vi "Referential Leaves to Objects.vi"(11 "Reference Items":T1(array[cluster])) -> (3 "Reference Objects":refnum<class "Referential.lvclass">[](array[class]))   [LabVIEW 2019, in "ParseGDSII.lvclass"]
uses:
  ParseGDSII.lvclass
  Elements/Referential.lvclass
  06f77329-d20e-40e9-99c9-cf91113c5fcf.vi/492f4e88-b7c6-4100-97d4-f1e35eb10a82.vi
  <vilib>/Utility/Debug Log/Display.vi
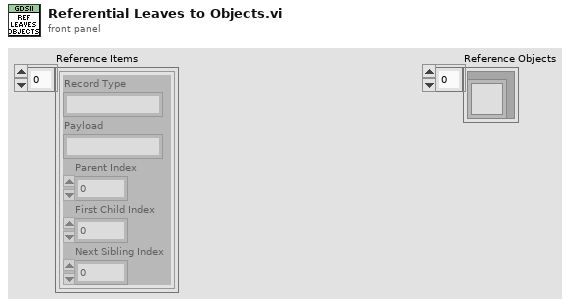
[diagram p1: front panel]
types:
  T1 = cluster{"Record Type":string, "Payload":string, "Parent Index":i32, "First Child Index":i32, "Next Sibling Index":i32}[]
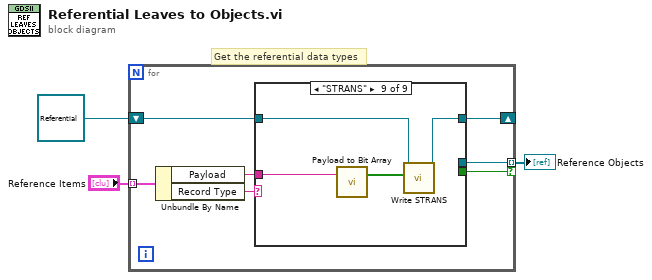
[diagram p0: block diagram]
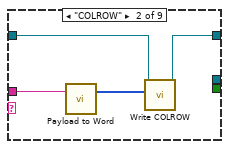
[diagram p3: hidden frame]
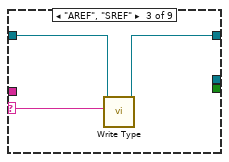
[diagram p4: hidden frame]
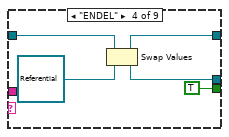
[diagram p5: hidden frame]
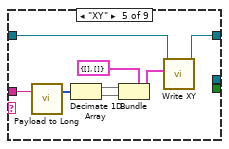
[diagram p6: hidden frame]
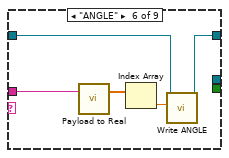
[diagram p7: hidden frame]
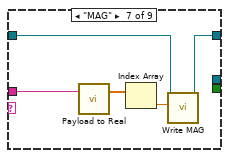
[diagram p8: hidden frame]
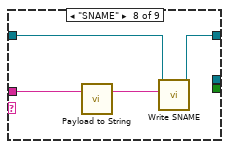
[diagram p9: hidden frame]
diagram:
  # "Get the referential data types"
  n1 = for {
    tunnel: "Reference Items" -> [w10] mode=indexing
    tunnel: [w5] -> w1 mode=indexing if=w4
    shift-right: [w7] -> _
    shift-left: refnum<class "Referential.lvclass"> refnum ("Referential.lvclass") -> [w6]
    n2 = Unbundle By Name(w10) -> ("Payload"=w9:string, "Record Type"=w8:string)
    n3 = case shown="\"STRANS\"" w8 {
      selector: w8 -> [_ _ w16 _ _ _ _ _ _]
      tunnel: w9 -> [_ w15 _ _ w26 w32 w40 w43 w47]
      tunnel: [w11 w12 w18 w20 w25 w35 w38 w45 w48] -> w7
      tunnel: w6 -> [w11 w13 w17 w21 w24 w36 w39 w44 w49]
      tunnel: [_ _ _ w22 _ _ _ _ _] -> w5
      tunnel: [_ _ _ TRUE _ _ _ _ _] -> w4
      frame Default {
      }
      frame "COLROW" {
        n4 = call "Payload to Word.vi"("Payload"=w15) -> ("Word"=w14:i16[])  [unwired: 2 in]
        n5 = call-dynamic "Write COLROW.vi"("COLROW"=w14, "Referential in"=w13) -> ("Referential out"=w12:refnum<class "Referential.lvclass">)  [unwired: 8 in, 1 out]
      }
      frame "AREF", "SREF" {
        n6 = call-dynamic "Write Type.vi"("Type"=w16, "Element in"=w17) -> ("Element out"=w18:refnum<class "Referential.lvclass">)  [unwired: 8 in, 1 out]
      }
      frame "ENDEL" {
        n7 = Swap Values(12:w21, 14:refnum<class "Referential.lvclass"> refnum ("Referential.lvclass")) -> (1:w20:refnum<class "Referential.lvclass">, 3:w22:refnum<class "Referential.lvclass">)  [unwired: 1 in]
      }
      frame "XY" {
        n8 = call "Payload to Long.vi"("Payload"=w26) -> ("Long"=w29:i32[])  [unwired: 2 in]
        n9 = Decimate 1D Array(w29) -> (w31:i32[], w30:i32[])
        n10 = Bundle(cluster=cluster{"X":i32[], "Y":i32[]} {"X"=[], "Y"=[]} ("XY"), "X"=w31, "Y"=w30) -> (w28:cluster{"X":i32[], "Y":i32[]})
        n11 = call-dynamic "Write XY.vi"("XY"=w28, "Element in"=w24) -> ("Element out"=w25:refnum<class "Referential.lvclass">)  [unwired: 8 in, 1 out]
      }
      frame "ANGLE" {
        n12 = call "Payload to Real.vi"("Payload"=w32) -> ("Real"=w33:dbl[])  [unwired: 2 in]
        n13 = Index Array(array=w33) -> (element=w34:dbl)  [unwired: 1 in]
        n14 = call-dynamic "Write ANGLE.vi"("ANGLE"=w34, "Referential in"=w36) -> ("Referential out"=w35:refnum<class "Referential.lvclass">)  [unwired: 8 in, 1 out]
      }
      frame "MAG" {
        n15 = call "Payload to Real.vi"("Payload"=w40) -> ("Real"=w41:dbl[])  [unwired: 2 in]
        n16 = Index Array(array=w41) -> (element=w37:dbl)  [unwired: 1 in]
        n17 = call-dynamic "Write MAG.vi"("MAG"=w37, "Referential in"=w39) -> ("Referential out"=w38:refnum<class "Referential.lvclass">)  [unwired: 8 in, 1 out]
      }
      frame "SNAME" {
        n18 = call "Payload to String.vi"("Payload"=w43) -> ("String"=w42:string)  [unwired: 2 in]
        n19 = call-dynamic "Write SNAME.vi"("SNAME"=w42, "Referential in"=w44) -> ("Referential out"=w45:refnum<class "Referential.lvclass">)  [unwired: 8 in, 1 out]
      }
      frame "STRANS" {
        n20 = call "Payload to Bit Array.vi"("Payload"=w47) -> ("Bit Array"=w46:bool[])  [unwired: 2 in]
        n21 = call-dynamic "Write STRANS.vi"("STRANS"=w46, "Referential in"=w49) -> ("Referential out"=w48:refnum<class "Referential.lvclass">)  [unwired: 8 in, 1 out]
      }
    }
  }
  "Reference Objects" <- w1
